vi "getEventForceActuatorInfo.vi"(11 "Publisher in":refnum<class "Publisher.lvclass">) -> (2 "EventForceActuatorInfo":T1, 3 "Publisher out":refnum<class "Publisher.lvclass">)   [LabVIEW 2016, in "Publisher.lvclass"]
uses:
  Publisher.lvclass
  DataTypes/Topics/EventForceActuatorInfo.ctl
  DataTypes/Topics/Parts/Timestamp.ctl
  Publisher.lvclass/Publisher.ctl
  DataTypes/Topics/M1M3SupportTopics.lvlib
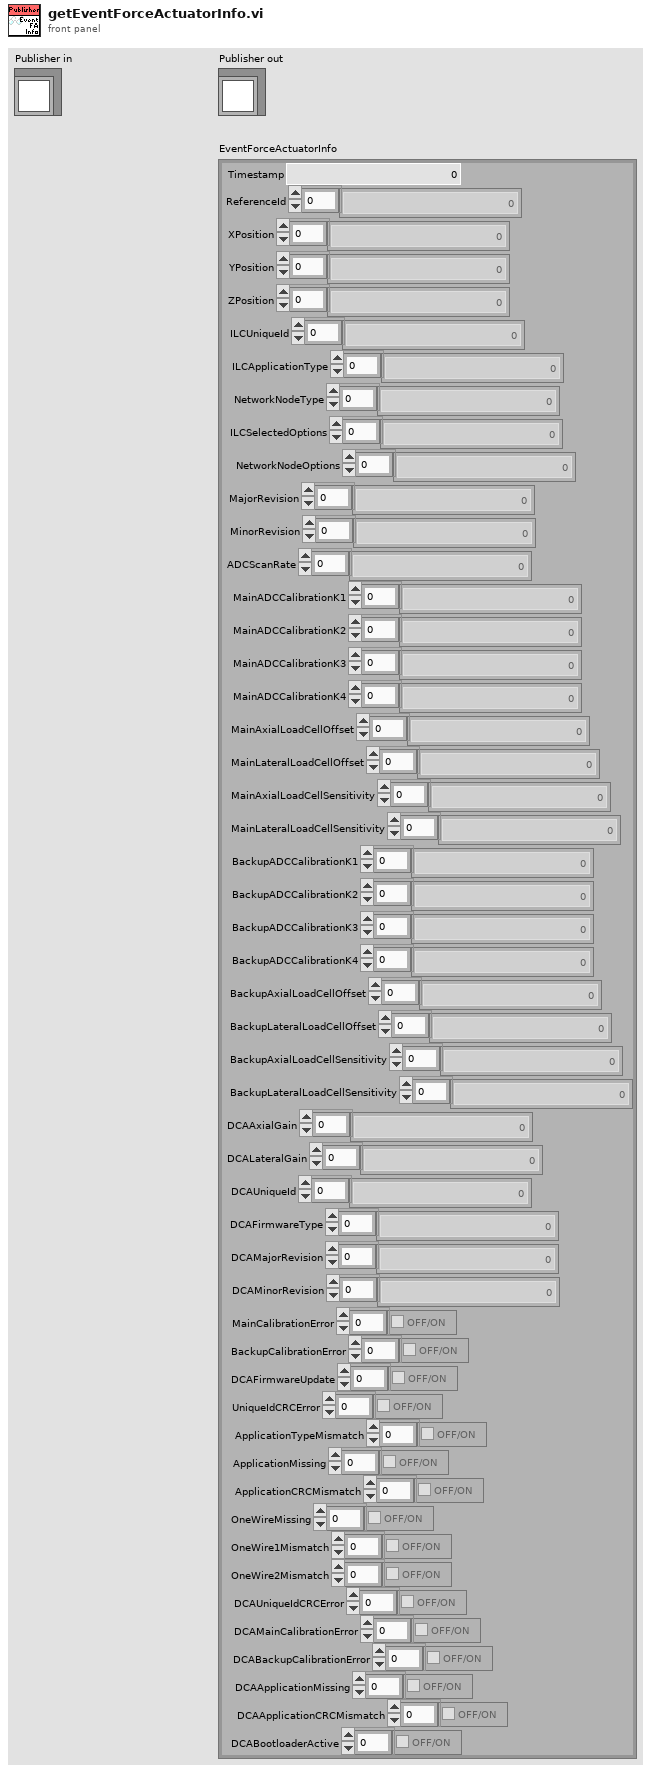
[diagram p1: front panel]
types:
  T1 = typedef "M1M3SupportTopics.lvlib/EventForceActuatorInfo.ctl" = cluster{"Timestamp":T2, "ReferenceId":i32[], "XPosition":sgl[], "YPosition":sgl[], "ZPosition":sgl[], "ILCUniqueId":i64[], "ILCApplicationType":u8[], "NetworkNodeType":u8[], "ILCSelectedOptions":u8[], "NetworkNodeOptions":u8[], "MajorRevision":u8[], "MinorRevision":u8[], "ADCScanRate":u8[], "MainADCCalibrationK1":sgl[], "MainADCCalibrationK2":sgl[], "MainADCCalibrationK3":sgl[], "MainADCCalibrationK4":sgl[], "MainAxialLoadCellOffset":sgl[], "MainLateralLoadCellOffset":sgl[], "MainAxialLoadCellSensitivity":sgl[], "MainLateralLoadCellSensitivity":sgl[], "BackupADCCalibrationK1":sgl[], "BackupADCCalibrationK2":sgl[], "BackupADCCalibrationK3":sgl[], "BackupADCCalibrationK4":sgl[], "BackupAxialLoadCellOffset":sgl[], "BackupLateralLoadCellOffset":sgl[], "BackupAxialLoadCellSensitivity":sgl[], "BackupLateralLoadCellSensitivity":sgl[], "DCAAxialGain":sgl[], "DCALateralGain":sgl[], "DCAUniqueId":i64[], "DCAFirmwareType":u8[], "DCAMajorRevision":u8[], "DCAMinorRevision":u8[], "MainCalibrationError":bool[], "BackupCalibrationError":bool[], "DCAFirmwareUpdate":bool[], "UniqueIdCRCError":bool[], "ApplicationTypeMismatch":bool[], "ApplicationMissing":bool[], "ApplicationCRCMismatch":bool[], "OneWireMissing":bool[], "OneWire1Mismatch":bool[], "OneWire2Mismatch":bool[], "DCAUniqueIdCRCError":bool[], "DCAMainCalibrationError":bool[], "DCABackupCalibrationError":bool[], "DCAApplicationMissing":bool[], "DCAApplicationCRCMismatch":bool[], "DCABootloaderActive":bool[]}
  T2 = typedef "M1M3SupportTopics.lvlib/Timestamp.ctl" = dbl
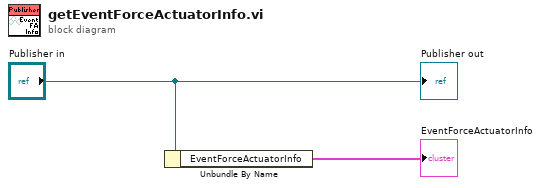
[diagram p0: block diagram]
diagram:
  n1 = Unbundle By Name("Publisher in") -> ("EventForceActuatorInfo"=→"EventForceActuatorInfo":T1)
  "Publisher out" <- "Publisher in"
